vi "p1.vi"() -> ()   [LabVIEW 2025, in "d6.lvlib"]
uses:
  d6.lvlib
  <vilib>/Utility/error.llb/Trim Whitespace One-Sided.vi
  AOC/AOC.lvlib
panel:
  in  "Example":string="123 328  51 64 \n 45 64  387 23 \n  6 98  215 314\n*   +   *   +  "
  in  "Example":bool=TRUE
  out "Answer":u64=1909
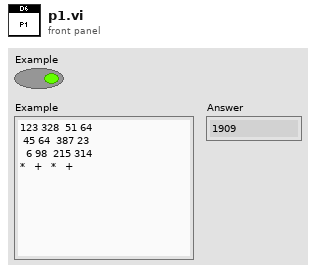
[diagram p1: front panel]
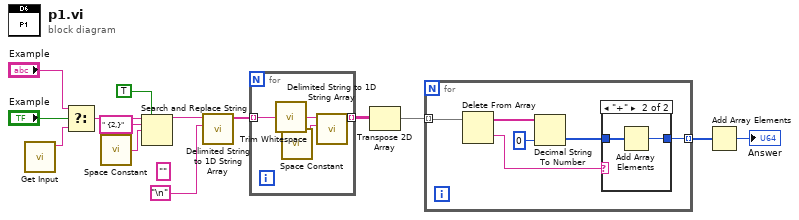
[diagram p0: block diagram]
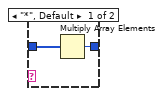
[diagram p2: hidden frame]
diagram:
  (unwired) "" ("format string")
  n1 = call "Get Input.vi"() -> ("Input"=w14:string)  [unwired: 11 in]
  n2 = Select(t="Example", s="Example", f=w14) -> (s? t:f=w8:string)
  n3 = call <vilib>:"Space Constant.vi"() -> ("String"=w5:string)
  n4 = Search and Replace String(replace all?=TRUE ("replace all? (F)"), input string=w8, search string=" {2,}", replace string=w5) -> (result string=w4:string)  [unwired: 4 in, 3 out]
  n5 = call <vilib>:"Delimited String to 1D String Array.vi"("delimiter"="\n", "delimited string"=w4) -> ("string array"=w2:string[])  [unwired: 9 in]
  n6 = for {
    tunnel: w2 -> [w18] mode=indexing
    tunnel: [w15] -> w1 mode=indexing
    n7 = call <vilib>:"Trim Whitespace.vi"("string"=w18) -> ("trimmed string"=w17:string)  [unwired: 1 in]
    n8 = call <vilib>:"Space Constant.vi"() -> ("String"=w16:string)
    n9 = call <vilib>:"Delimited String to 1D String Array.vi"("delimiter"=w16, "delimited string"=w17) -> ("string array"=w15:string[])  [unwired: 9 in]
  }
  n10 = Transpose 2D Array(2D array=w1) -> (transposed array=w11:string[][])
  n11 = for {
    tunnel: w11 -> [w24] mode=indexing
    tunnel: [w20] -> w10 mode=indexing
    n12 = Delete From Array(array=w24) -> (deleted portion=w21:string, array with subset deleted=w23:string[])  [unwired: 2 in]
    n13 = Decimal String To Number(string=w23, default (0L)=u64 0 ("default (0 I32)")) -> (number=w22:u64[])  [unwired: 1 in, 1 out]
    n14 = case shown="\"+\"" w21 {
      tunnel: w22 -> [w26 w28]
      tunnel: [w25 w27] -> w20
      frame "*", Default {
        n15 = Multiply Array Elements(1:w26) -> (0:w25:u64)
      }
      frame "+" {
        n16 = Add Array Elements(numeric array=w28) -> (sum=w27:u64)
      }
    }
  }
  n17 = Add Array Elements(numeric array=w10) -> (sum=→"Answer":u64)
